vi "SVN_Log_ParseOutput.vi"() -> ()   [LabVIEW 2014]
uses:
  <vilib>/xml/NI_XML.lvlib
  <resource>/objmgr/DOMUserDefRef.rc
  <vilib>/xml/Load XML File.vi
panel:
  out "Value":string[](array[string])
  out "XML PP":string
  out "node Name":string
  out "logentry Name":string
  out "Node Value":string
  out "Name":string[](array[string])
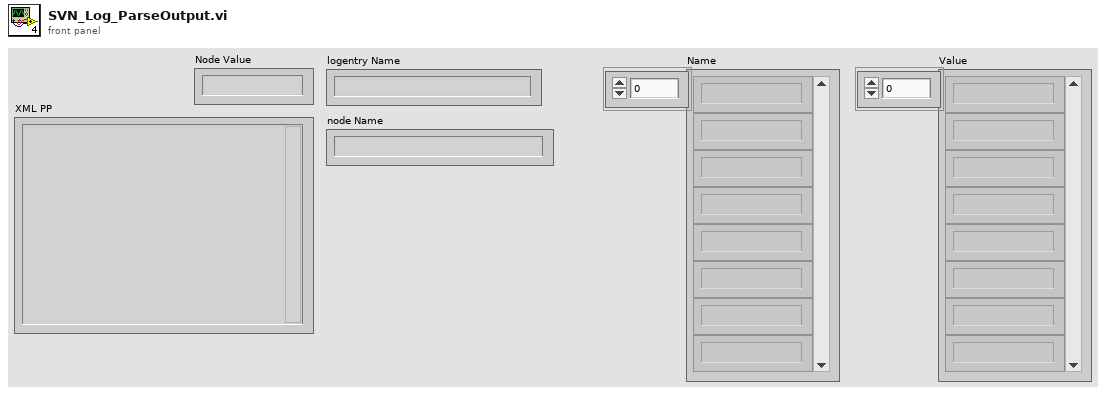
[diagram p1: front panel]
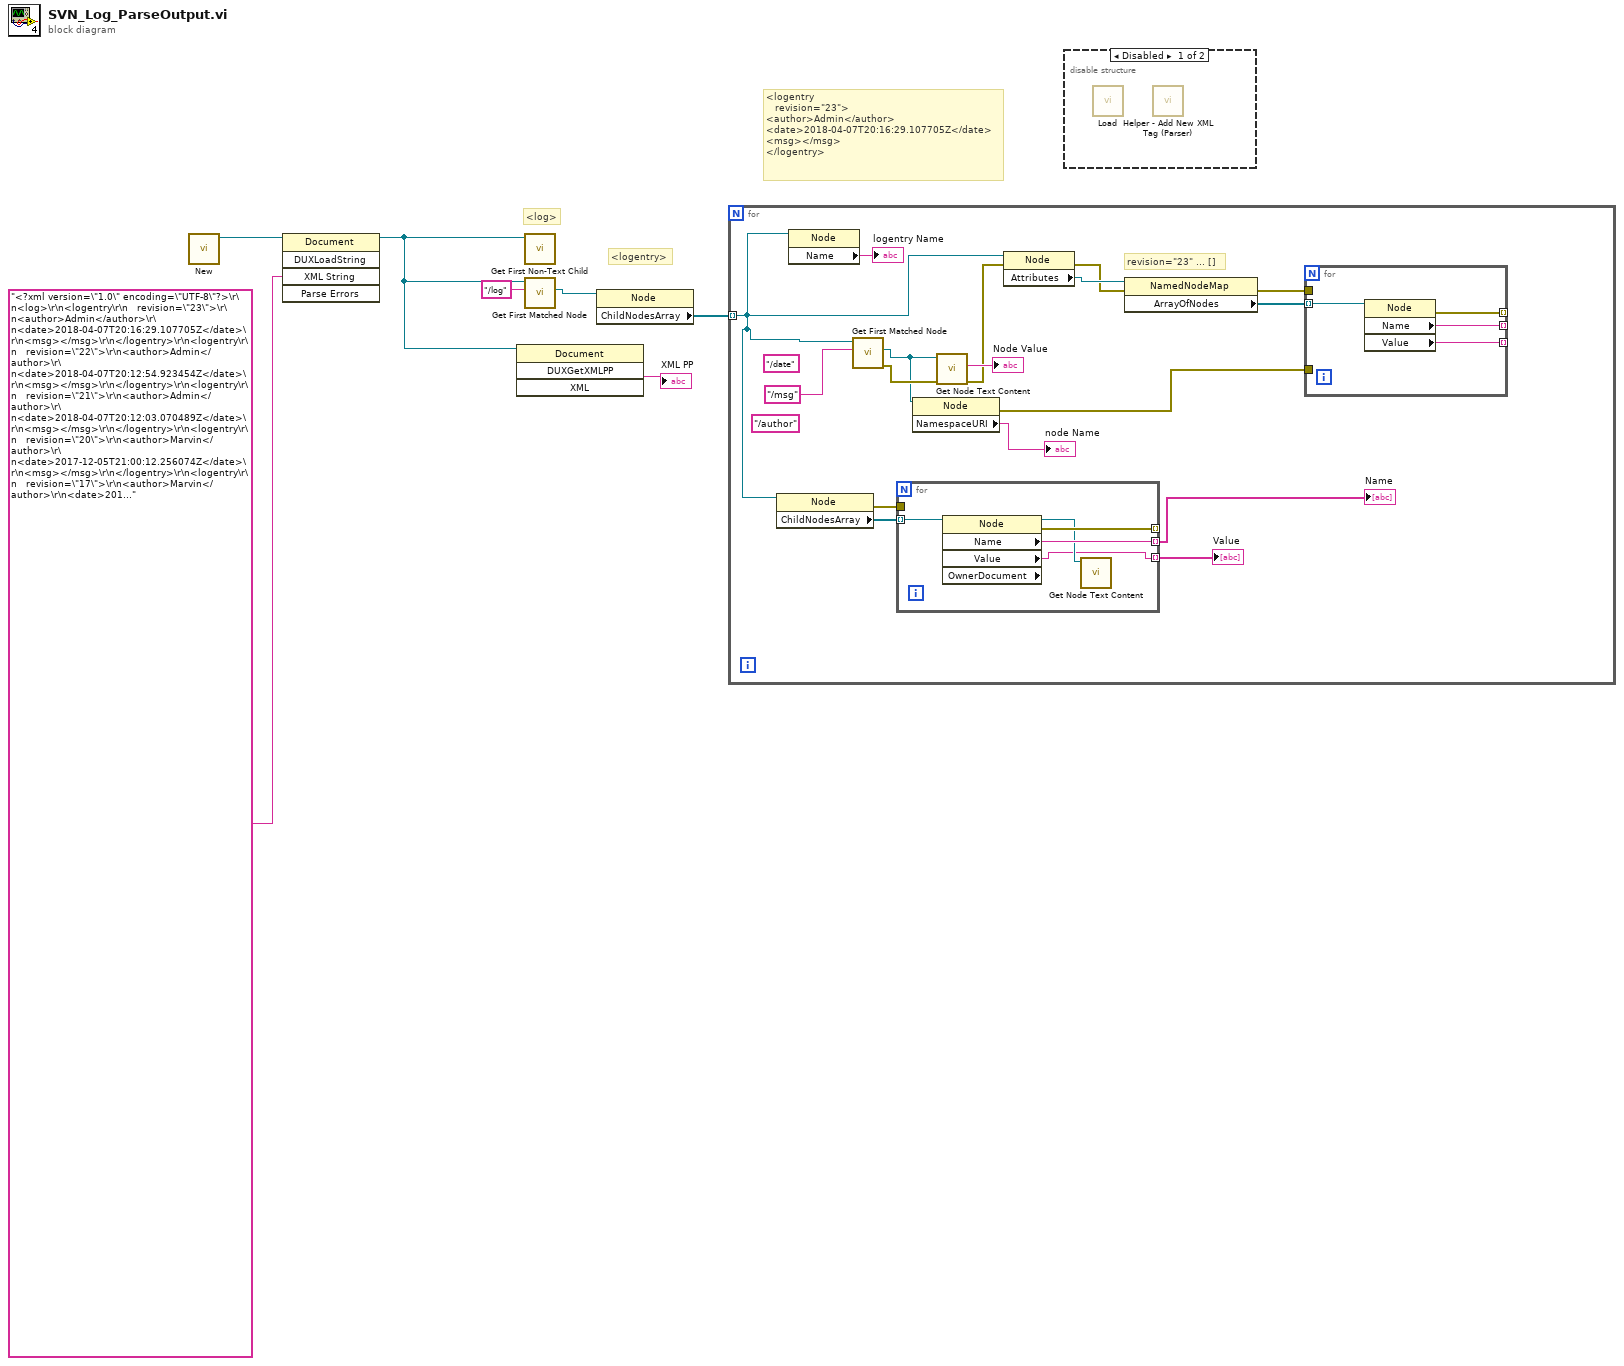
[diagram p0: block diagram]
diagram:
  # "<logentry\n   revision=\"23\">\n<author>Admin</author>\n<date>2018-04-07T20:16:29.107705Z</date>\n<msg></msg>\n</logentry>"
  # "<logentry>"
  # "<log>"
  n1 = call <vilib>:"New.vi"() -> ("DOM document out"=w7:refnum<k20>)  [unwired: 8 in, 1 out]
  n2 = invoke class="Document" method="DUXLoadString"(reference=w7, "XML String"="<?xml version=\"1.0\" encoding=\"UTF-8\"?>\r\n<log>\r\n<logentry\r\n   revision=\"23\">\r\n<author>Admin</author>\r\n<date>2018-04-07T20:16:29.107705Z</date>\r\n<msg></msg>\r\n</logentry>\r\n<logentry\r\n   revision=\"22\">\r\n<author>Admin</author>\r\n<date>2018-04-07T20:12:54.923454Z</date>\r\n<msg></msg>\r\n</logentry>\r\n<logentry\r\n   revision=\"21\">\r\n<author>Admin</author>\r\n<date>2018-04-07T20:12:03.070489Z</date>\r\n<msg></msg>\r\n</logentry>\r\n<logentry\r\n   revision=\"20\">\r\n<author>Marvin</author>\r\n<date>2017-12-05T21:00:12.256074Z</date>\r\n<msg></msg>\r\n</logentry>\r\n<logentry\r\n   revision=\"17\">\r\n<author>Marvin</author>\r\n<date>2017-12-05T20:36:10.326601Z</date>\r\n<msg>10k LoadSpeedTest\r\n</msg>\r\n</logentry>\r\n<logentry\r\n   revision=\"16\">\r\n<author>Marvin</author>\r\n<date>2017-07-06T14:47:03.129259Z</date>\r\n<msg></msg>\r\n</logentry>\r\n<logentry\r\n   revision=\"11\">\r\n<author>Marvin</author>\r\n<date>2017-07-04T16:12:46.837966Z</date>\r\n<msg></msg>\r\n</logentry>\r\n<logentry\r\n   revision=\"7\">\r\n<author>Marvin</author>\r\n<date>2017-07-04T16:05:39.382517Z</date>\r\n<msg></msg>\r\n</logentry>\r\n<logentry\r\n   revision=\"6\">\r\n<author>Marvin</author>\r\n<date>2017-07-04T16:05:05.356571Z</date>\r\n<msg></msg>\r\n</logentry>\r\n<logentry\r\n   revision=\"3\">\r\n<author>Marvin</author>\r\n<date>2017-07-04T15:57:28.132419Z</date>\r\n<msg></msg>\r\n</logentry>\r\n<logentry\r\n   revision=\"1\">\r\n<author>Marvin</author>\r\n<date>2017-07-04T15:51:57.071483Z</date>\r\n<msg>Imported folder structure</msg>\r\n</logentry>\r\n</log>\r\n" ("standard output")) -> (reference out=w1:refnum<k20>)  [unwired: 3 in, 4 out]
  n3 = invoke class="Document" method="DUXGetXMLPP"(reference=w1) -> ("XML"=→"XML PP":string)  [unwired: 3 in, 3 out]
  n4 = call <vilib>:"Get First Non-Text Child.vi"("node in"=w1) -> ()  [unwired: 7 in, 4 out]
  n5 = call <vilib>:"Get First Matched Node.vi"("XPath expression"="/log", "node in"=w1) -> ("node result"=w2:refnum<k20>)  [unwired: 7 in, 2 out]
  n6 = property class="Node"(reference=w2) -> ("ChildNodesArray"=w5:refnum<k20>[])  [unwired: 1 in, 2 out]
  n7 = for {
    tunnel: w5 -> [w12] mode=indexing
    (unwired) "/author" ("XPath expression")
    (unwired) "/date" ("XPath expression")
    # "revision=\"23\" ... []"
    n8 = property class="Node"(reference=w12) -> (error out=w10:errorcluster, "ChildNodesArray"=w11:refnum<k20>[])  [unwired: 1 in, 1 out]
    n9 = property class="Node"(reference=w12) -> ("Name"=→"logentry Name":string)  [unwired: 1 in, 2 out]
    n10 = call <vilib>:"Get First Matched Node.vi"("XPath expression"="/msg", "node in"=w12) -> ("error out"=w18:errorcluster, "node result"=w15:refnum<k20>)  [unwired: 7 in, 1 out]
    n11 = for {
      tunnel: w11 -> [w29] mode=indexing
      tunnel: [w25] -> w8 mode=indexing
      tunnel: [w28] -> _ mode=indexing
      tunnel: [w27] -> w9 mode=indexing
      tunnel: w10 -> [_]
      n12 = property class="Node" props=["Name", "Value", "OwnerDocument"](reference=w29) -> (reference out=w26:refnum<k20>, error out=w28:errorcluster, "Name"=w27:string, "Value"=w25:string)  [unwired: 1 in, 1 out]
      n13 = call <vilib>:"Get Node Text Content.vi"("node in"=w26) -> ()  [unwired: 8 in, 3 out]
    }
    "Name" <- w9
    "Value" <- w8
    n14 = property class="Node"(reference=w15) -> (error out=w14:errorcluster, "NamespaceURI"=→"node Name":string)  [unwired: 1 in, 1 out]
    n15 = call <vilib>:"Get Node Text Content.vi"("error in (no error)"=w18, "node in"=w15) -> ("error out"=w17:errorcluster, "node text"=→"Node Value":string)  [unwired: 7 in, 1 out]
    n16 = property class="Node"(reference=w12, error in=w17) -> (error out=w21:errorcluster, "Attributes"=w24:refnum<k20>)  [unwired: 1 out]
    n17 = property class="NamedNodeMap"(reference=w24, error in=w21) -> (error out=w22:errorcluster, "ArrayOfNodes"=w23:refnum<k20>[])  [unwired: 1 out]
    n18 = for {
      tunnel: w23 -> [w33] mode=indexing
      tunnel: [w32] -> _ mode=indexing
      tunnel: w22 -> [_]
      tunnel: [w31] -> _ mode=indexing
      tunnel: [w30] -> _ mode=indexing
      tunnel: w14 -> [_]
      n19 = property class="Node"(reference=w33) -> (error out=w31:errorcluster, "Name"=w30:string, "Value"=w32:string)  [unwired: 1 in, 1 out]
    }
  }
  n20 = disable-structure shown="Disabled" {
    frame Disabled {
      n21 = call-poly <vilib>:"Load.vi"() -> ()  [unwired: 13 in, 3 out]
      n22 = call "Helper - Add New XML Tag (Parser).vi"() -> ()  [unwired: 9 in, 3 out]
    }
    frame Enabled {
    }
  }
